vi "AK Logger.vi"   [LabVIEW 2020, in "AK-Schnittstelle.lvlib"]
uses:
  AK-Schnittstelle.lvlib
  Aktionen Gespeicherte Werte.ctl
  Daten weitergeben Aktionen.ctl
  Allgemein/allgemeine Sub-VIs.lvlib
panel:
  # "AK Kommunikation in Datei loggen!"
types:
  T1 = typedef "AK-Schnittstelle.lvlib/Aktionen Gespeicherte Werte.ctl" = enum16{"lesen", "laden", "speichern", "Seriell", "TCP", "Diverse", "AKTIV", "AK-Namen"}
  T2 = typedef "AK-Schnittstelle.lvlib/Daten weitergeben Aktionen.ctl" = enum16{"lesen", "schreiben", "Log löschen", "Detail", "Detail löschen", "Speicher Freigeben"}
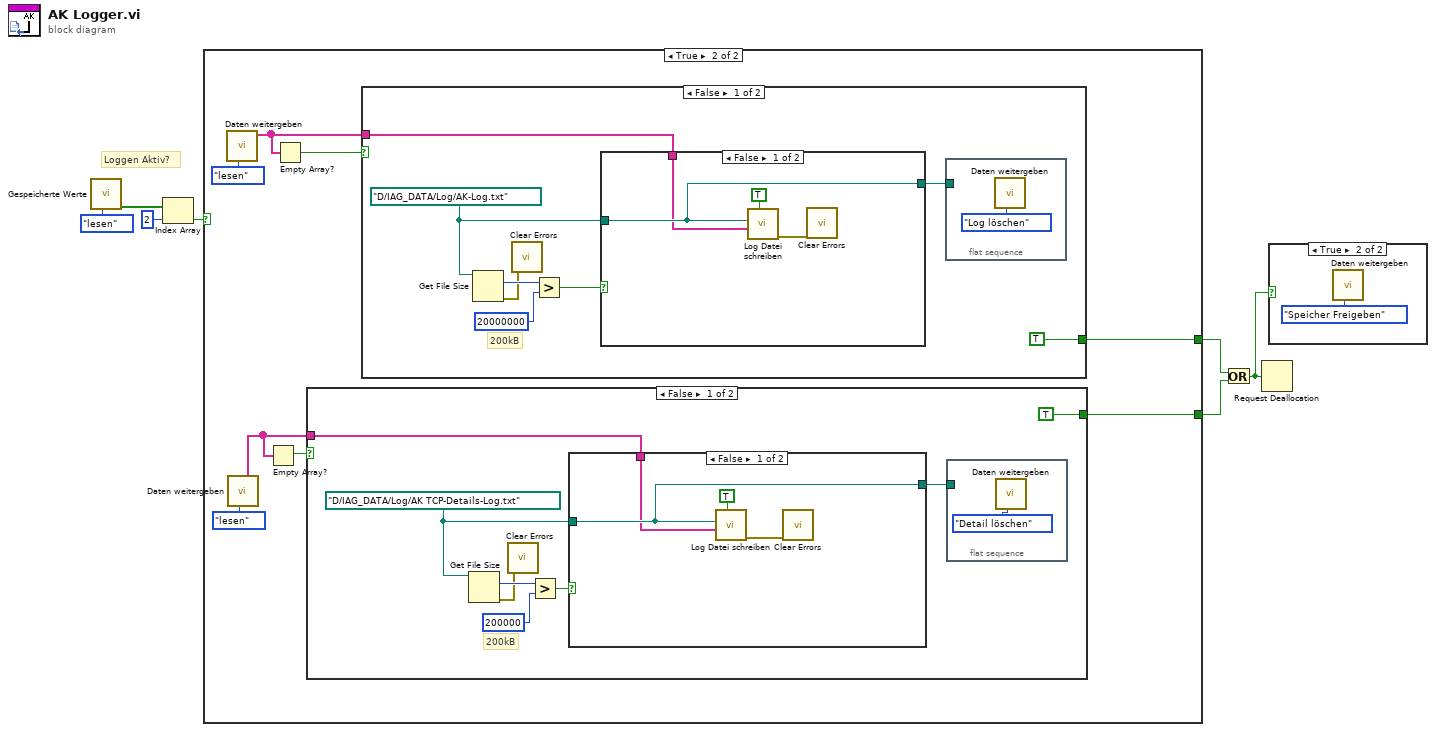
[diagram p0: block diagram]
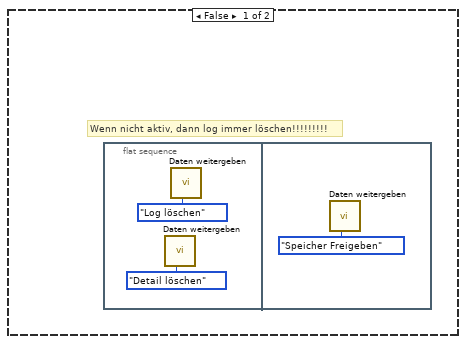
[diagram p3: hidden frame]
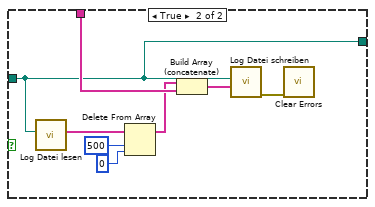
[diagram p4: hidden frame]
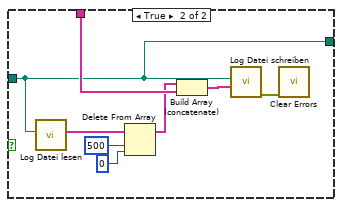
[diagram p6: hidden frame]
diagram:
  # "Loggen Aktiv?"
  n1 = call "Gespeicherte Werte.vi"("Aktionen"=Aktionen_Gespeicherte_Werte."lesen") -> ("AKTIV?"=w6:bool[])  [unwired: 6 in, 4 out]
  n2 = Index Array(array=w6, index=2 ("Index")) -> (element=w4:bool)
  n3 = case shown="True" w4 {
    tunnel: [_ w12] -> w2
    tunnel: [_ w11] -> w3
    frame False {
      # "Wenn nicht aktiv, dann log immer löschen!!!!!!!!!"
      n4 = flat-sequence {
        frame #0 {
          n5 = call "Daten weitergeben.vi"("Aktionen"=Daten_weitergeben_Aktionen."Detail löschen") -> ()  [unwired: 6 in, 5 out]
          n6 = call "Daten weitergeben.vi"("Aktionen"=Daten_weitergeben_Aktionen."Log löschen") -> ()  [unwired: 6 in, 5 out]
        }
        frame #1 {
          n7 = call "Daten weitergeben.vi"("Aktionen"=Daten_weitergeben_Aktionen."Speicher Freigeben") -> ()  [unwired: 6 in, 5 out]
        }
      }
    }
    frame True {
      n8 = call "Daten weitergeben.vi"("Aktionen"=Daten_weitergeben_Aktionen."lesen") -> ("Log Daten"=w17:string[])  [unwired: 6 in, 4 out]
      n9 = call "Daten weitergeben.vi"("Aktionen"=Daten_weitergeben_Aktionen."lesen") -> ("Details"=w14:string[])  [unwired: 6 in, 4 out]
      n10 = Empty Array?(array=w14) -> (empty?=w13:bool)
      n11 = Empty Array?(array=w17) -> (empty?=w16:bool)
      n12 = case shown="False" w13 {
        tunnel: w14 -> [w21 _]
        tunnel: [TRUE _] -> w12
        frame False {
          w23 = path "D:/IAG_DATA/Log/AK TCP-Details-Log.txt" ("Datei")
          # "200kB"
          n13 = Get File Size(file=w23) -> (size (in bytes)=w24:i64, 0:w22:errorcluster)  [unwired: 1 in, 1 out]
          n14 = call <vilib>:"Clear Errors.vi"("error in (no error)"=w22) -> ()  [unwired: 5 in, 2 out]
          n15 = Greater?(x=w24, y=i64 200000) -> (0:w26:bool)
          n16 = case shown="False" w26 {
            tunnel: w21 -> [w29 w37]
            tunnel: w23 -> [w30 w34]
            tunnel: [w30 w34] -> w20
            frame False {
              n17 = call "Log Datei schreiben.vi"("An Datei Anhängen?"=TRUE, "Array"=w29, "Dateipfad"=w30) -> ("error out"=w28:errorcluster)  [unwired: 8 in]
              n18 = call <vilib>:"Clear Errors.vi"("error in (no error)"=w28) -> ()  [unwired: 5 in, 2 out]
            }
            frame True {
              n19 = call "Log Datei lesen.vi"("Dateipfad"=w34) -> ("Array"=w35:string[])  [unwired: 10 in]
              n20 = Delete From Array(array=w35, length=500 ("Länge"), index=0 ("Index")) -> (array with subset deleted=w36:string[])  [unwired: 1 out]
              n21 = Build Array (concatenate)(w36, w37) -> (w32:string[])
              n22 = call "Log Datei schreiben.vi"("Array"=w32, "Dateipfad"=w34) -> ("error out"=w33:errorcluster)  [unwired: 9 in]
              n23 = call <vilib>:"Clear Errors.vi"("error in (no error)"=w33) -> ()  [unwired: 5 in, 2 out]
            }
          }
          n24 = flat-sequence {
            tunnel: w20 -> [_]
            frame #0 {
              n25 = call "Daten weitergeben.vi"("Aktionen"=Daten_weitergeben_Aktionen."Detail löschen") -> ()  [unwired: 6 in, 5 out]
            }
          }
        }
        frame True {
        }
      }
      n26 = case shown="False" w16 {
        tunnel: w17 -> [w42 _]
        tunnel: [TRUE _] -> w11
        frame False {
          w44 = path "D:/IAG_DATA/Log/AK-Log.txt" ("Datei")
          # "200kB"
          n27 = Get File Size(file=w44) -> (size (in bytes)=w45:i64, 0:w43:errorcluster)  [unwired: 1 in, 1 out]
          n28 = call <vilib>:"Clear Errors.vi"("error in (no error)"=w43) -> ()  [unwired: 5 in, 2 out]
          n29 = Greater?(x=w45, y=i64 20000000) -> (0:w47:bool)
          n30 = case shown="False" w47 {
            tunnel: w42 -> [w50 w58]
            tunnel: w44 -> [w51 w55]
            tunnel: [w51 w55] -> w41
            frame False {
              n31 = call "Log Datei schreiben.vi"("An Datei Anhängen?"=TRUE, "Array"=w50, "Dateipfad"=w51) -> ("error out"=w49:errorcluster)  [unwired: 8 in]
              n32 = call <vilib>:"Clear Errors.vi"("error in (no error)"=w49) -> ()  [unwired: 5 in, 2 out]
            }
            frame True {
              n33 = call "Log Datei lesen.vi"("Dateipfad"=w55) -> ("Array"=w56:string[])  [unwired: 10 in]
              n34 = Delete From Array(array=w56, length=500 ("Länge"), index=0 ("Index")) -> (array with subset deleted=w57:string[])  [unwired: 1 out]
              n35 = Build Array (concatenate)(w57, w58) -> (w54:string[])
              n36 = call "Log Datei schreiben.vi"("Array"=w54, "Dateipfad"=w55) -> ("error out"=w53:errorcluster)  [unwired: 9 in]
              n37 = call <vilib>:"Clear Errors.vi"("error in (no error)"=w53) -> ()  [unwired: 5 in, 2 out]
            }
          }
          n38 = flat-sequence {
            tunnel: w41 -> [_]
            frame #0 {
              n39 = call "Daten weitergeben.vi"("Aktionen"=Daten_weitergeben_Aktionen."Log löschen") -> ()  [unwired: 6 in, 5 out]
            }
          }
        }
        frame True {
        }
      }
    }
  }
  n40 = Or(x=w3, y=w2) -> (x .or. y?=w1:bool)
  n41 = Request Deallocation(w1) -> ()
  n42 = case shown="True" w1 {
    frame False {
    }
    frame True {
      n43 = call "Daten weitergeben.vi"("Aktionen"=Daten_weitergeben_Aktionen."Speicher Freigeben") -> ()  [unwired: 6 in, 5 out]
    }
  }
